vi "GlyphIndexPairs.vi"(7 "action":T1, 8 "error in":errorcluster, 9 "array":T2[](array[typedef]), 10 "glyph":string) -> (0 "error out":errorcluster, 2 "index":i32)   [LabVIEW 2013, in "NISE_CEF_TreeControl.lvlib"]
doc: "This VI creates a list of Glyph name and index pairs. It will be used to retrieve Glyphs by name. Glyphs are case sensitive. If the Glyph is not found it returns an Warning saying Glyph not found"
uses:
  NISE_CEF_TreeControl.lvlib
  Controls/GlyphIndexPair.ctl
  Controls/GlyphIndexPairActions.ctl
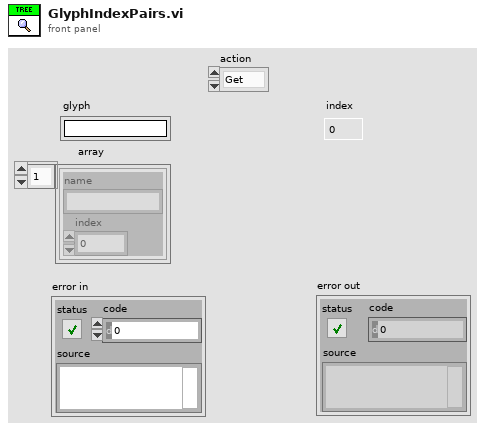
[diagram p1: front panel]
types:
  T1 = typedef "NISE_CEF_TreeControl.lvlib/GlyphIndexPairActions.ctl" = enum16{"Get", "Initialize"}
  T2 = typedef "NISE_CEF_TreeControl.lvlib/GlyphIndexPair.ctl" = cluster{"name":string, "index":i32}
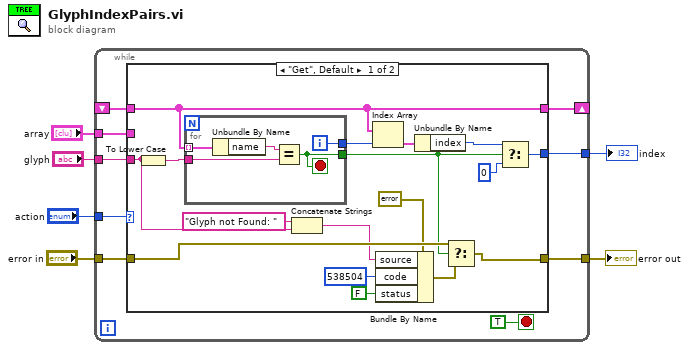
[diagram p0: block diagram]
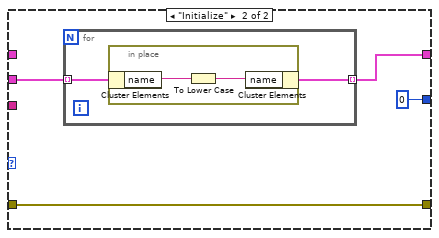
[diagram p2: hidden frame]
diagram:
  n1 = while {
    tunnel: "glyph" -> [w15]
    tunnel: [w14] -> w5
    shift-right: [w11] -> _
    shift-left: _ -> [w12]
    tunnel: "array" -> [w10]
    tunnel: "action" -> [w9]
    tunnel: "error in" -> [w8]
    tunnel: [w7] -> w1
    stop <- TRUE stop-if-true
    n2 = case shown="\"Get\", Default" w9 {
      tunnel: w15 -> [w19 _]
      tunnel: [w29 0 ("f")] -> w14
      tunnel: w12 -> [w27 _]
      tunnel: [w27 w38] -> w11
      tunnel: w10 -> [_ w39]
      tunnel: w8 -> [w26 w40]
      tunnel: [w25 w40] -> w7
      frame "Get", Default {
        n3 = To Lower Case(string=w19) -> (all lower case string=w20:string)
        n4 = for {
          tunnel: w27 -> [w37] mode=indexing
          tunnel: w20 -> [w36]
          tunnel: [w34] -> w32
          tunnel: [w33] -> w21
          i -> [w34]
          stop <- w33 stop-if-true
          n5 = Unbundle By Name(w37) -> ("name"=w35:string)
          n6 = Equal?(x=w35, y=w36) -> (x = y?=w33:bool)
        }
        n7 = Concatenate Strings("Glyph not Found: " ("string"), w19) -> (w22:string)
        n8 = Index Array(array=w27, index=w32) -> (element=w28:T2)
        n9 = Bundle By Name(cluster=errorcluster {"status"=FALSE, "code"=0, "source"=""} ("error in"), "source"=w22, "code"=538504, "status"=FALSE) -> (w16:errorcluster)
        n10 = Unbundle By Name(w28) -> ("index"=w31:i32)
        n11 = Select(t=w26, s=w21, f=w16) -> (s? t:f=w25:errorcluster)
        n12 = Select(t=w31, s=w21, f=0) -> (s? t:f=w29:i32)
      }
      frame "Initialize" {
        n13 = for {
          tunnel: w39 -> [w43] mode=indexing
          tunnel: [w42] -> w38 mode=indexing
          n14 = in-place {
            n15 = in-place-cluster #1(w43) -> ("name"=w45:string)
            n16 = To Lower Case(string=w45) -> (all lower case string=w44:string)
            n17 = in-place-cluster #1("name"=w44) -> (w42:T2)
          }
        }
      }
    }
  }
  "index" <- w5
  "error out" <- w1
